vi "pulse 488 and steady 594.vi"(9 "594 amplitude":dbl=1.0 format="%0.2f", 11 "488 nm channel parameters":T1={"voltage"=0.0, "frequency"=0.0, "duty cycle"=0.0, "sample rate"=1000.0}) -> (3 "waveforms out":waveform(dbl)[](array[waveform]))   [LabVIEW 2025]
uses:
  channel parameters cluster.ctl
  <vilib>/Waveform/WDTOps.llb/WDT Number of Waveform Samples DBL.vi
  <vilib>/Analysis/NI_AALBase.lvlib
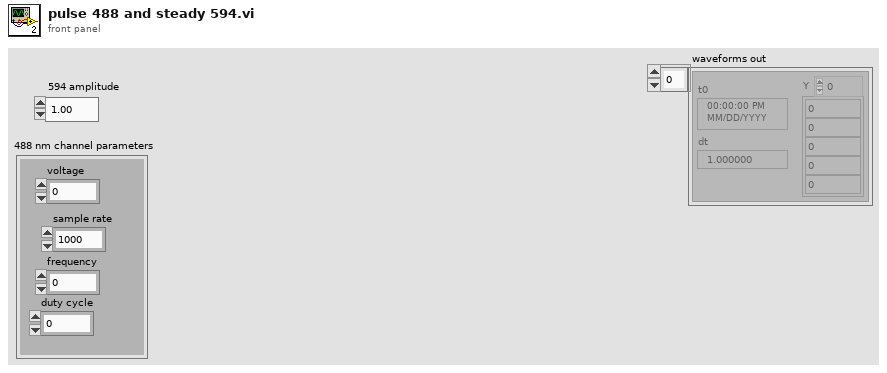
[diagram p1: front panel]
types:
  T1 = typedef "channel parameters cluster.ctl" = cluster{"voltage":dbl, "frequency":dbl, "duty cycle":dbl, "sample rate":dbl}
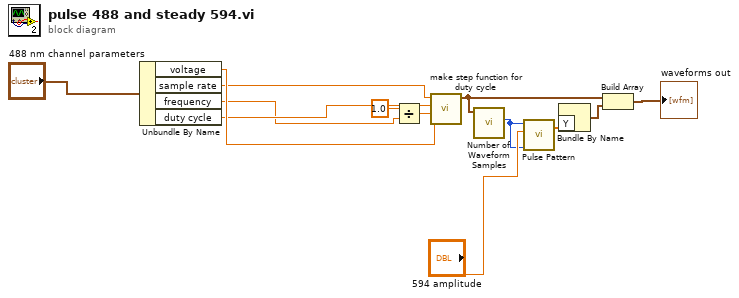
[diagram p0: block diagram]
diagram:
  n1 = Unbundle By Name("488 nm channel parameters") -> ("voltage"=w5:dbl, "sample rate"=w4:dbl, "frequency"=w2:dbl, "duty cycle"=w3:dbl)
  n2 = Divide(x=1.0, y=w2) -> (x/y=w12:dbl)
  n3 = call "make step function for duty cycle.vi"("amplitude"=w5, "period"=w12, "duty cycle"=w3, "sample rate"=w4) -> ("Waveform out"=w11:waveform(dbl))  [unwired: 7 in]
  n4 = call-poly <vilib>:"Number of Waveform Samples.vi"("waveform in"=w11) -> ("number of samples"=w7:i32)  [unwired: 8 in, 2 out]
  n5 = call <vilib>:"Pulse Pattern.vi"("width"=w7, "amplitude"="594 amplitude", "samples"=w7) -> ("Pulse Pattern"=w9:dbl[])  [unwired: 1 in, 1 out]
  n6 = Bundle By Name("Y"=w9) -> (w8:waveform(dbl))  [unwired: 1 in]
  n7 = Build Array(w11, w8) -> (→"waveforms out":waveform(dbl)[])
